vi "GUI.DAQmxName.Get.vi"(8 "error in (no error)":errorcluster, 11 "deviceDAQName":string) -> (0 "error out":errorcluster, 2 "DeviceDAQConnect":tag)   [LabVIEW 2019]
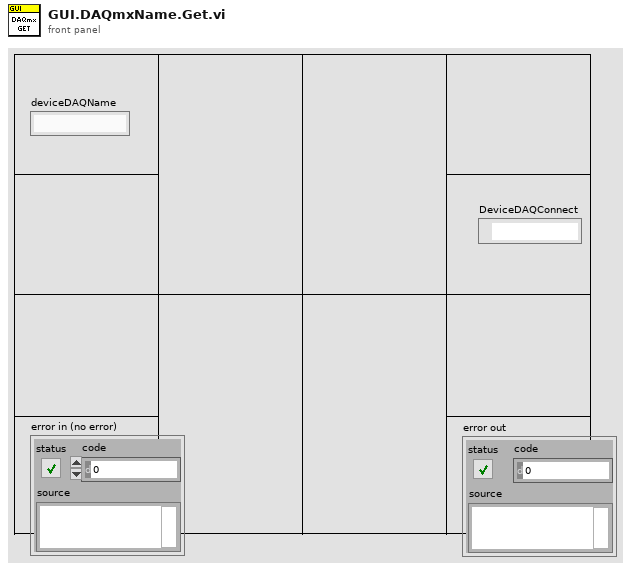
[diagram p1: front panel]
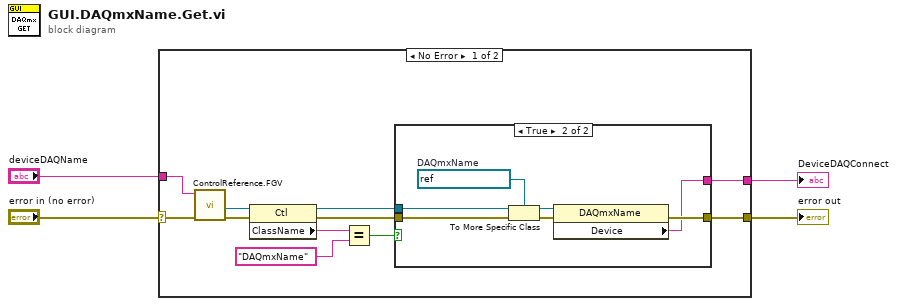
[diagram p0: block diagram]
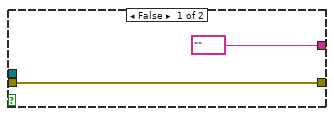
[diagram p2: hidden frame]
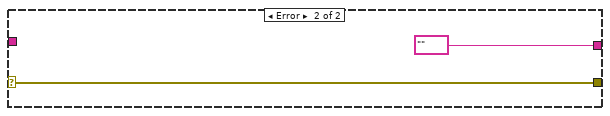
[diagram p3: hidden frame]
diagram:
  n1 = case shown="No Error" "error in (no error)" {
    selector: "error in (no error)" -> [w15 w26]
    tunnel: [w10 w26] -> w3
    tunnel: "deviceDAQName" -> [w6 _]
    tunnel: [w5 tag "" ("Device")] -> w4
    frame No Error {
      n2 = call "ControlReference.FGV.vi"("error in (no error)"=w15, "controlLabelText"=w6) -> ("error out"=w14:errorcluster, "referenceToControl"=w13:refnum<vi>)  [unwired: 8 in]
      n3 = property class="Ctl"(reference=w13, error in=w14) -> (reference out=w9:refnum<vi>, error out=w11:errorcluster, "ClassName"=w12:string)
      n4 = Equal?(x=w12, y="DAQmxName") -> (x = y?=w8:bool)
      n5 = case shown="True" w8 {
        tunnel: w11 -> [w17 w24]
        tunnel: [w17 w19] -> w10
        tunnel: w9 -> [_ w23]
        tunnel: [tag "" ("Device") w18] -> w5
        frame False {
        }
        frame True {
          w22 = refnum<vi> refnum  # DAQmxName
          n6 = To More Specific Class(target class=w22, reference=w23, error in=w24) -> (specific class reference=w21:refnum<vi>, error out=w20:errorcluster)
          n7 = property class="DAQmxName"(reference=w21, error in=w20) -> (error out=w19:errorcluster, "Device"=w18:tag)  [unwired: 1 out]
        }
      }
    }
    frame Error {
    }
  }
  "DeviceDAQConnect" <- w4
  "error out" <- w3
